vi "DB Path.vi"() -> (3 "DB path":path)   [LabVIEW 2020, in "Settings.lvlib"]
uses:
  Settings.lvlib
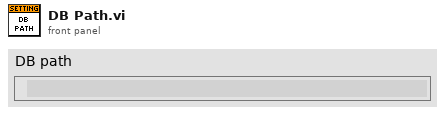
[diagram p1: front panel]
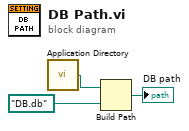
[diagram p0: block diagram]
diagram:
  n1 = call <vilib>:"Application Directory.vi"() -> ("Application Directory"=w1:path)
  n2 = Build Path(base path=w1, name or relative path=path "DB.db" ("base path")) -> (appended path=→"DB path":path)
